vi "Build FIlters.vi"() -> ()   [LabVIEW 2011]
uses:
  <vilib>/addons/Digital Filter Design/_Objects.llb/DFD Quantization Settings.ctl
  <vilib>/addons/Digital Filter Design/_Objects.llb/DFD Quantization Sources.ctl
  <vilib>/addons/Digital Filter Design/_Objects.llb/DFD Round-off Mode.ctl
  <vilib>/addons/Digital Filter Design/_Objects.llb/DFD Output Iwl Obj.ctl
  <vilib>/addons/Digital Filter Design/_Objects.llb/DFD Coef Norm Type.ctl
  <vilib>/Utility/file.llb/Write To Spreadsheet File (DBL).vi
  <vilib>/addons/Digital Filter Design/FXPModel.llb/DFD FXP Quantize Coef (Advanced).vi
  <vilib>/addons/Digital Filter Design/NI_DigFilterLicensed.lvlib
panel:
  in  "path":path=path "R:/Troca/danielot/Davi/Corr2"
  out "mSRate_QCoef.gain":dbl
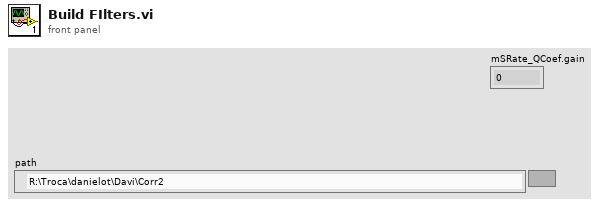
[diagram p1: front panel]
types:
  T1 = cluster{"gain":dbl, "zeroes":cdb[], "poles":cdb[]}[][]
  T2 = typedef "NI_DigFilterLicensed.lvlib/DFD Quantization Settings.ctl" = cluster{"source":T3, "wl":i16, "iwl":i16, "overflow mode":enum16{"Saturation", "Wrap"}, "rounding mode":enum16{"Nearest", "Truncation"}, "signed?":bool}
  T3 = typedef "NI_DigFilterLicensed.lvlib/DFD Quantization Sources.ctl" = u16
  T4 = typedef "NI_DigFilterLicensed.lvlib/DFD Round-off Mode.ctl" = enum16{"Nearest", "Truncation"}
  T5 = typedef "NI_DigFilterLicensed.lvlib/DFD Output Iwl Obj.ctl" = cluster{"output option":enum16{"Auto", "Same As Input", "User Defined"}, "integer word length":i16}
  T6 = typedef "NI_DigFilterLicensed.lvlib/DFD Coef Norm Type.ctl" = enum16{"No Norm", "Time Domain 1-Norm", "Time Domain 2-Norm", "Time Domain Inf-Norm"}
  T7 = typedef "NI_DigFilterLicensed.lvlib/DFD Filter Obj.ctl" = cluster{"mSRate_Fs":dbl, "mSRate_Version":string, "mSRate_Comments":string, "mSRate_OrgCoef":T8, "mSRate_CurCoef":T8, "mSRate_Quantized?":bool, "mSRate_QCoef":T8, "mSRate_QSettings":T10[], "mSRate_Order":i32, "mSRate_Scaling":cluster{"mSRate_ScaleByPowerOf2?":bool, "mSRate_ScaleType":T6}}
  T8 = typedef "NI_DigFilterLicensed.lvlib/DFD Filter Coef.ctl" = cluster{"type":T9, "gain":dbl, "coef a (k)":dbl[], "coef b (v)":dbl[]}
  T9 = typedef "NI_DigFilterLicensed.lvlib/DFD Filter Structure Type Selector.ctl" = enum16{"Undefined", "FIR Direct Form", "FIR Direct Form Transposed", "FIR Symmetric", "FIR Antisymmetric", "IIR Direct Form I", "IIR Direct Form I Transposed", "IIR Direct Form II", "IIR Direct Form II Transposed", "IIR Cascaded Second Order Sections Form I", "IIR Cascaded Second Order Sections Form I Transposed", "IIR Cascaded Second Order Sections Form II", "IIR Cascaded Second Order Sections Form II Transposed", "Lattice Allpass (basic sections)", "Lattice Allpass (one multiplier sections)", "Lattice Allpass (normalized sections)", "Lattice AR (basic sections)", "Lattice AR (one multiplier sections)", "Lattice AR (normalized sections)", "Lattice MA (minimum phase)", "Lattice MA (maximum phase)", "Lattice ARMA (basic sections)", "Lattice ARMA (one multiplier sections)", "Lattice ARMA (normalized sections)"}
  T10 = typedef "NI_DigFilterLicensed.lvlib/dfd_Internal Quantization Settings.ctl" = cluster{"source":T11, "wl":i16, "iwl":i16, "overflow mode":enum16{"Saturation", "Wrap"}, "rounding mode":enum16{"Nearest", "Truncation"}, "signed?":bool}
  T11 = typedef "NI_DigFilterLicensed.lvlib/dfd_Internal Quantization Srcs.ctl" = u16
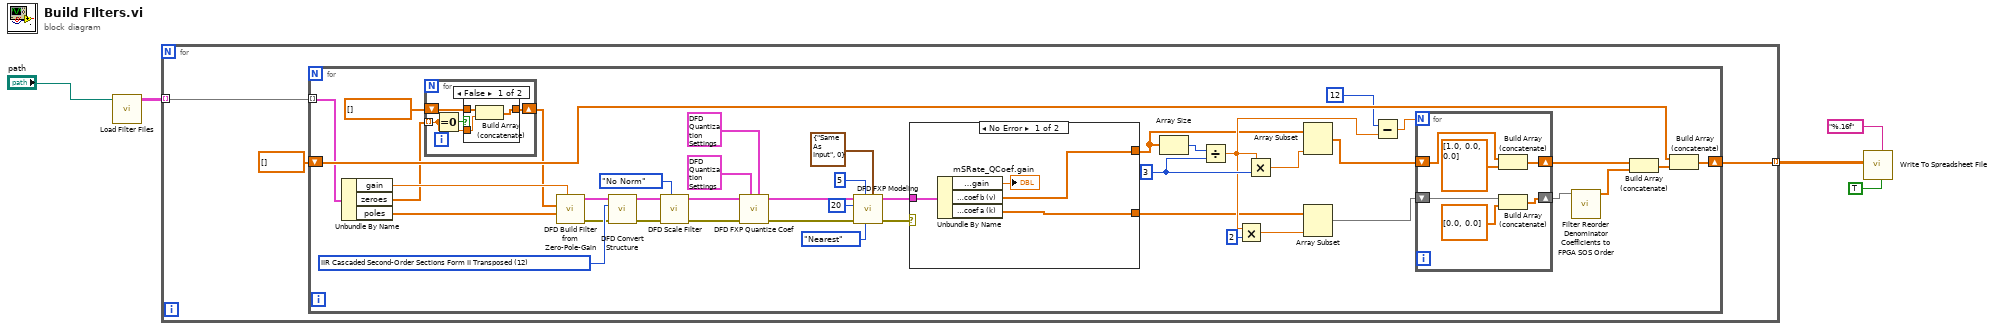
[diagram p0: block diagram]
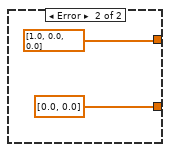
[diagram p3: hidden frame]
diagram:
  n1 = call "Load Filter Files.vi"("path"="path") -> ("Array of Filters"=w4:T1)  [unwired: 10 in]
  n2 = for {
    tunnel: [w7] -> w3 mode=indexing
    tunnel: w4 -> [w6] mode=indexing
    n3 = for {
      shift-right: [w49] -> w7
      shift-left: dbl[] [] -> [w48]
      tunnel: w6 -> [w26] mode=indexing
      w34 = u16 12 items=["FIR Direct Form"=1, "FIR Direct Form Transposed"=2, "FIR Symmetric"=3, "FIR Antisymmetric"=4, "IIR Direct Form I"=5, "IIR Direct Form I Transposed"=6, "IIR Direct Form II"=7, "IIR Direct Form II Transposed"=8, "IIR Cascaded Second-Order Sections Form I"=9, "IIR Cascaded Second-Order Sections Form I Transposed"=10, "IIR Cascaded Second-Order Sections Form II"=11, "IIR Cascaded Second-Order Sections Form II Transposed"=12, "Lattice Allpass (basic sections)"=13, "Lattice Allpass (one multiplier sections)"=14, "Lattice Allpass (normalized sections)"=15, "Lattice AR (basic sections)"=16, "Lattice AR (one multiplier sections)"=17, "Lattice AR (normalized sections)"=18, "Lattice MA (minimum phase)"=19, "Lattice MA (maximum phase)"=20, "Lattice ARMA (basic sections)"=21, "Lattice ARMA (one multiplier sections)"=22, "Lattice ARMA (normalized sections)"=23] ("target structure")
      w37 = 3 ("y")
      n4 = Unbundle By Name(w26) -> ("gain"=w24:dbl, "zeroes"=w11:cdb[], "poles"=w25:cdb[])
      n5 = for {
        tunnel: w11 -> [w52] mode=indexing
        shift-right: [w51] -> w9
        shift-left: cdb[] [] ("zeroes") -> [w53]
        n6 = Equal To 0?(x=w52) -> (x = 0?=w54:bool)
        n7 = case shown="False" w54 {
          tunnel: w53 -> [w57 w58]
          tunnel: [w56 w58] -> w51
          tunnel: w52 -> [w55 _]
          frame False {
            n8 = Build Array (concatenate)(w57, w55) -> (w56:cdb[])
          }
          frame True {
          }
        }
      }
      n9 = call <vilib>:"DFD Build Filter from Zero-Pole-Gain.vi"("gain"=w24, "poles"=w25, "zeroes"=w9) -> ("error out"=w29:errorcluster, "filter out"=w30:T7)  [unwired: 7 in]
      n10 = call <vilib>:"DFD Convert Structure.vi"("error in (no error)"=w29, "target structure"=w34, "filter in"=w30) -> ("error out"=w32:errorcluster, "filter out"=w31:T7)  [unwired: 7 in]
      n11 = call <vilib>:"DFD Scale Filter.vi"("scale type"=DFD_Coef_Norm_Type."No Norm", "error in (no error)"=w32, "filter in"=w31) -> ("error out"=w16:errorcluster, "filter out"=w15:T7)  [unwired: 7 in]
      n12 = call-poly <vilib>:"DFD FXP Quantize Coef.vi"("coefficients b/v quantizer"=T2 {"source"=7, "wl"=22, "iwl"=4, "overflow mode"=enum."Saturation", "rounding mode"=enum."Nearest", "signed?"=TRUE}, "coefficients a/k quantizer"=T2 {"source"=0, "wl"=22, "iwl"=4, "overflow mode"=enum."Saturation", "rounding mode"=enum."Nearest", "signed?"=TRUE}, "error in (no error)"=w16, "filter in"=w15) -> ("error out"=w18:errorcluster, "filter out"=w14:T7)  [unwired: 6 in]
      n13 = call <vilib>:"DFD FXP Modeling.vi"("output integer word length"=T5 {"output option"=enum."Same As Input", "integer word length"=0}, "output rounding mode"=DFD_Round-off_Mode."Nearest", "input integer word length"=i16 5, "error in (no error)"=w18, "input word length"=i16 20, "filter in"=w14) -> ("error out"=w12:errorcluster, "filter out"=w13:T7)  [unwired: 4 in]
      n14 = case shown="No Error" w12 {
        tunnel: [w62 dbl[] [1.0, 0.0, 0.0] ("coef b (v)")] -> w28
        tunnel: [w61 dbl[] [0.0, 0.0] ("coef a (k)")] -> w27
        tunnel: w13 -> [w60 _]
        frame No Error {
          n15 = Unbundle By Name(w60) -> ("mSRate_QCoef.gain"=→"mSRate_QCoef.gain":dbl, "mSRate_QCoef.coef b (v)"=w62:dbl[], "mSRate_QCoef.coef a (k)"=w61:dbl[])
        }
        frame Error {
        }
      }
      n16 = Array Size(array=w28) -> (size(s)=w35:i32)
      n17 = Divide(x=w35, y=w37) -> (x/y=w36:dbl)
      n18 = Multiply(x=w36, y=2) -> (x*y=w41:dbl)
      n19 = Multiply(x=w36, y=w37) -> (x*y=w42:dbl)
      n20 = Array Subset(array=w28, length=w42) -> (w43:dbl[])  [unwired: 1 in]
      n21 = Array Subset(array=w27, length=w41) -> (w40:dbl[])  [unwired: 1 in]
      n22 = Subtract(x=12, y=w36) -> (x-y=w38:dbl)
      n23 = for {
        N: w38 -> [_]
        shift-right: [w68] -> w47
        shift-left: w43 -> [w70]
        shift-right: [w65] -> w46
        shift-left: w40 -> [w67]
        n24 = Build Array (concatenate)(w70, dbl[] [1.0, 0.0, 0.0]) -> (w68:dbl[])
        n25 = Build Array (concatenate)(w67, dbl[] [0.0, 0.0]) -> (w65:dbl[])
      }
      n26 = call "Filter Reorder Denominator Coefficients to FPGA SOS Order.vi"("coef a (k)"=w46) -> ("coef a (k)"=w45:dbl[])  [unwired: 10 in]
      n27 = Build Array (concatenate)(w47, w45) -> (w50:dbl[])
      n28 = Build Array (concatenate)(w48, w50) -> (w49:dbl[])
    }
  }
  n29 = call-poly <vilib>:"Write To Spreadsheet File.vi"("transpose? (no:F)"=TRUE, "format (%.3f)"="%.16f", "2D data"=w3) -> ()  [unwired: 5 in, 1 out]
